vi "stft_demodulate.vi"(6 "STFT params":T1={"Win param"=120.0, "Window type"=102, "Win order"=8, "DFT size"=64, "Channels"=[7], "Oversample"=64} {"Oversample" min=1 step=1; "Channels" min=0 step=1; "DFT size" min=1 step=1; "Window type" items=["Rectangle"=0, "Hanning"=1, "Hamming"=2, "Blackman-Harris"=3, "Exact Blackman"=4, "Blackman"=5, "Flat Top"=6, "4 Term B-Harris "=7, "7 Term B-Harris"=8, "Low Sidelobe"=9, "Blackman Nuttall"=11, "Triangle"=30, "Bartlett-Hanning"=31, "Bohman"=32, "Parzen"=33, "Welch"=34, "Kaiser"=60, "Dolph-Chebyshev"=61, "Gaussian"=62]}, 8 "Reset":bool, 10 "X":dbl[](array[numeric])) -> (0 "error out":errorcluster, 1 "time-freq sample info":cluster{"time steps":i32, "frequency bins":i32}, 3 "STFT":cdb[][](array[numeric]))   [LabVIEW 2026]
uses:
  stft_params.ctl
  <vilib>/Analysis/4window.llb/windowTd.ctl
  <vilib>/Analysis/NI_AALPro.lvlib
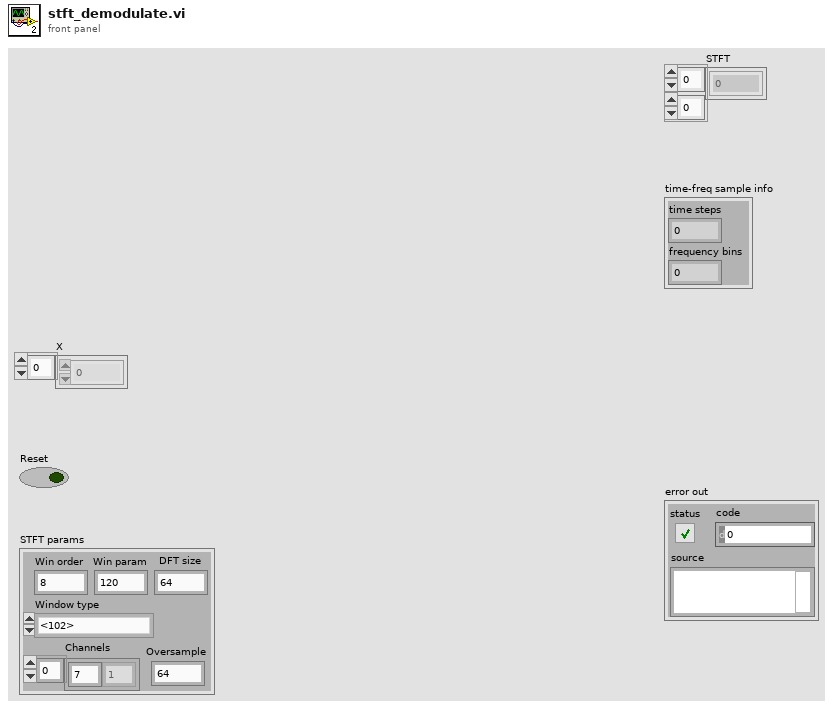
[diagram p1: front panel]
types:
  T1 = typedef "stft_params.ctl" = cluster{"Win param":dbl, "Window type":T2, "Win order":i32, "DFT size":i32, "Channels":i32[], "Oversample":i32}
  T2 = typedef "NI_AALPro.lvlib/windowTd.ctl" = u32
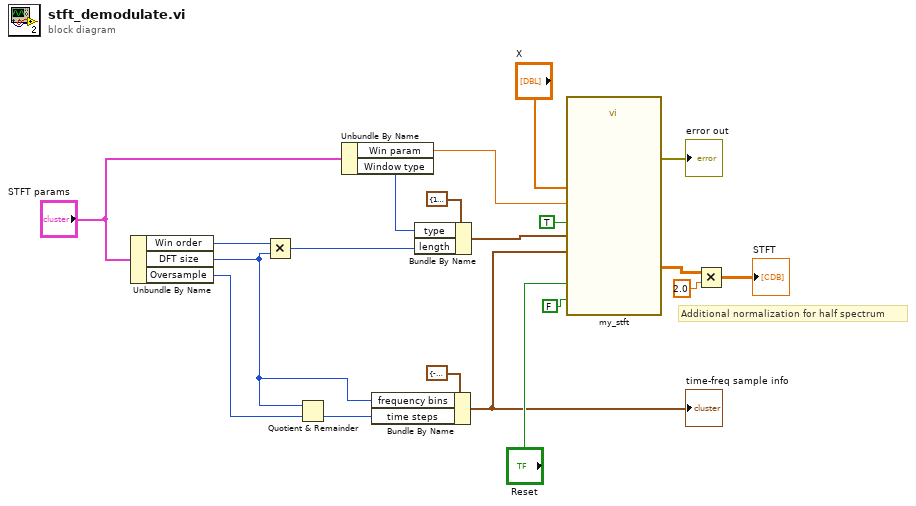
[diagram p0: block diagram]
diagram:
  # "Additional normalization for half spectrum"
  n1 = Unbundle By Name("STFT params") -> ("Win order"=w9:i32, "DFT size"=w7:i32, "Oversample"=w6:i32)
  n2 = Multiply(x=w9, y=w7) -> (x*y=w13:i32)
  n3 = Quotient & Remainder(x=w7, y=w6) -> (floor(x/y)=w5:i32)  [unwired: 1 out]
  n4 = Unbundle By Name("STFT params") -> ("Win param"=w11:dbl, "Window type"=w10:T2)
  n5 = Bundle By Name(cluster=cluster{"time steps":i32, "frequency bins":i32} {"time steps"=-1, "frequency bins"=512} ("time-freq sampling info"), "frequency bins"=w7, "time steps"=w5) -> (w12:cluster{"time steps":i32, "frequency bins":i32})
  "time-freq sample info" <- w12
  n6 = Bundle By Name(cluster=cluster{"type":T2, "length":i32} {"type"=1, "length"=64} ("window info"), "type"=w10, "length"=w13) -> (w18:cluster{"type":T2, "length":i32})
  n7 = call "my_stft.vi"("Reset"="Reset", "FFT normalize"=TRUE, "force freq bins to power of 2?"=FALSE, "window parameter"=w11, "window info"=w18, "time-freq sampling info"=w12, "X"="X") -> ("error out"=→"error out":errorcluster, "STFT {X}"=w4:cdb[][])  [unwired: 3 in]
  n8 = Multiply(x=w4, y=2.0 ("Win param")) -> (x*y=→"STFT":cdb[][])
